vi "checkValue.vi"(8 "Value":u32, 9 "Array of valid Values":u32[](array[numeric])) -> (3 "new Value":u32)   [LabVIEW 2013, in "Burst.lvclass"]
uses:
  Burst.lvclass
panel:
  out "index":i32
  in  "minDistance":i32
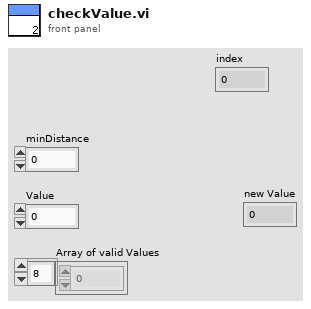
[diagram p1: front panel]
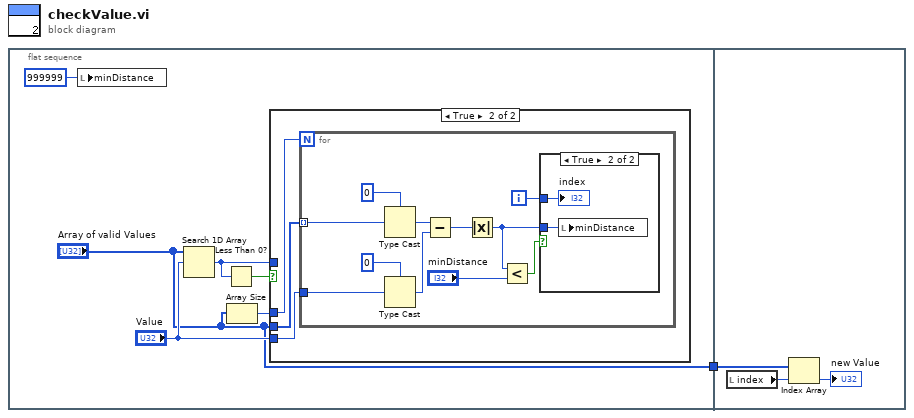
[diagram p0: block diagram]
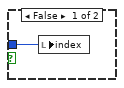
[diagram p2: hidden frame]
diagram:
  n1 = flat-sequence {
    tunnel: ["Array of valid Values"] -> w1
    tunnel: w1 -> [w26]
    frame #0 {
      n2 = local write "minDistance"(999999 ("minDistance")) -> ()
      n3 = Search 1D Array(1D array="Array of valid Values", element="Value") -> (index of element=w4:i32)  [unwired: 1 in]
      n4 = Less Than 0?(x=w4) -> (x < 0?=w5:bool)
      n5 = Array Size(array="Array of valid Values") -> (size(s)=w6:i32)
      n6 = case shown="True" w5 {
        tunnel: w6 -> [_ w11]
        tunnel: "Array of valid Values" -> [_ w10]
        tunnel: "Value" -> [_ w9]
        tunnel: w4 -> [w8 _]
        frame False {
          n7 = local write "index"(w8) -> ()
        }
        frame True {
          n8 = for {
            N: w11 -> [_]
            tunnel: w10 -> [w18] mode=indexing
            tunnel: w9 -> [w15]
            i -> [w22]
            n9 = Type Cast(type=0, x=w18) -> (*(type *) &x=w17:i32)
            n10 = Type Cast(type=0, x=w15) -> (*(type *) &x=w14:i32)
            n11 = Subtract(x=w17, y=w14) -> (x-y=w13:i32)
            n12 = Absolute Value(x=w13) -> (abs(x)=w12:i32)
            n13 = Less?(x=w12, y="minDistance") -> (x < y?=w20:bool)
            n14 = case shown="True" w20 {
              tunnel: w12 -> [_ w23]
              tunnel: w22 -> [_ w24]
              frame False {
              }
              frame True {
                n15 = local write "minDistance"(w23) -> ()
                "index" <- w24
              }
            }
          }
        }
      }
    }
    frame #1 {
      n16 = local read "index"() -> (w27:i32)
      n17 = Index Array(array=w26, index=w27) -> (element=→"new Value":u32)
    }
  }
